vi "Untitled 2.vi"() -> ()   [LabVIEW 2016]
uses:
  Classes/Controller/Motion/A3200/A3200.lvclass
panel:
  in  "XY":dbl[](array[numeric])
  in  "Speed":dbl
  in  "Numeric":dbl
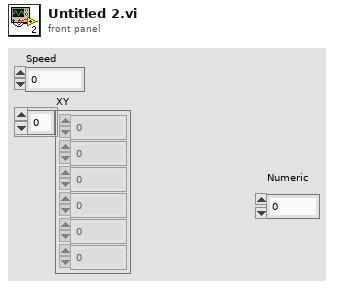
[diagram p1: front panel]
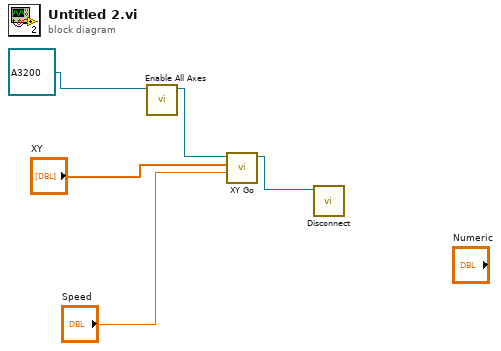
[diagram p0: block diagram]
diagram:
  n1 = call-dynamic "Enable All Axes.vi"("A3200 in"=refnum<class "A3200.lvclass"> refnum ("A3200.lvclass")) -> ("A3200 out"=w4:refnum<class "A3200.lvclass">)  [unwired: 9 in, 1 out]
  n2 = call-dynamic "XY Go.vi"("Speed"="Speed", "XY"="XY", "Gantry in"=w4) -> ("Gantry out"=w1:refnum<class "A3200.lvclass">)  [unwired: 7 in, 1 out]
  n3 = call-dynamic "Disconnect.vi"("Gantry in"=w1) -> ()  [unwired: 9 in, 1 out]
